vi "ObjectsClusterToArray-1.vi"(1 "[IN] Objects":T1(array[cluster]) {"Aspect Ratio" format="%.2f"; "Orientation" format="%.2f"; "Area" format="%.2f"; "Object Center"."Y" format="%.2f"; "Object Center"."X" format="%.2f"}) -> (0 "[OUT] X,Y Coordinates":dbl[](array[numeric]))   [LabVIEW 2020]
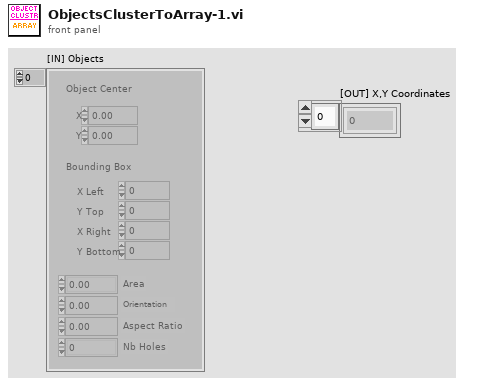
[diagram p1: front panel]
types:
  T1 = cluster{"Object Center":cluster{"X":sgl, "Y":sgl}, "Bounding Box":cluster{"X Left":i32, "Y Top":i32, "X Right":i32, "Y Bottom":i32}, "Area":sgl, "Orientation":sgl, "Aspect Ratio":sgl, "Nb Holes":i32}[]
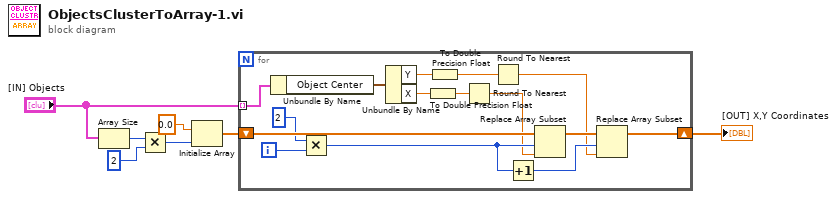
[diagram p0: block diagram]
diagram:
  n1 = Array Size(array="[IN] Objects") -> (size(s)=w6:i32)
  n2 = Multiply(x=w6, y=2) -> (x*y=w4:i32)
  n3 = Initialize Array(0.0 ("element"), w4) -> (w3:dbl[])
  n4 = for {
    tunnel: "[IN] Objects" -> [w13] mode=indexing
    shift-right: [w16] -> w2
    shift-left: w3 -> [w22]
    i -> [w21]
    n5 = Unbundle By Name(w13) -> ("Object Center"=w12:cluster{"X":sgl, "Y":sgl})
    n6 = Multiply(x=2 ("y"), y=w21) -> (x*y=w19:i32)
    n7 = Unbundle By Name(w12) -> ("Y"=w9:sgl, "X"=w10:sgl)
    n8 = To Double Precision Float(number=w10) -> (double precision float=w11:dbl)
    n9 = To Double Precision Float(number=w9) -> (double precision float=w8:dbl)
    n10 = Round To Nearest(number=w11) -> (nearest integer value=w15:dbl)
    n11 = Round To Nearest(number=w8) -> (nearest integer value=w14:dbl)
    n12 = Increment(x=w19) -> (x+1=w17:i32)
    n13 = Replace Array Subset(array=w22, new element=w15, index=w19) -> (w18:dbl[])
    n14 = Replace Array Subset(array=w18, new element=w14, index=w17) -> (w16:dbl[])
  }
  "[OUT] X,Y Coordinates" <- w2
